vi "Data Processor.vi"(8 "error in (no error)":errorcluster, 11 "Message Queues out":T1) -> (0 "error out":errorcluster, 3 "Message Queue":refnum<queue>)   [LabVIEW 2014]
uses:
  support/Message Queue/All Message Queues.ctl
  support/Message Queue/Message Cluster.ctl
  Data Processor cluster.ctl
  I Adj Parameters.ctl
  Engine/Message.ctl
  Teszt/Teszt.ctl
  Teszt/Command.ctl
  Analog/Enum AO.ctl
  Analog/Enum AI.ctl
  Digital/Enum DO.ctl
  <vilib>/Analysis/baseanly.llb/Mean (DBL).vi
  support/Message Queue/Enqueue Message (Single).vi
  global/Global 1.vi
  <vilib>/Utility/error.llb/Error Cluster From Error Code.vi
  <vilib>/ErrorRing/Error Ring.xnode
  support/Message Queue/Message Queue.lvlib
  Analog/Analog Input Cluster.ctl
  Analog/Analog Result Cluster.ctl
  Analog/Analog data.ctl
  <vilib>/Analysis/NI_AALBase.lvlib
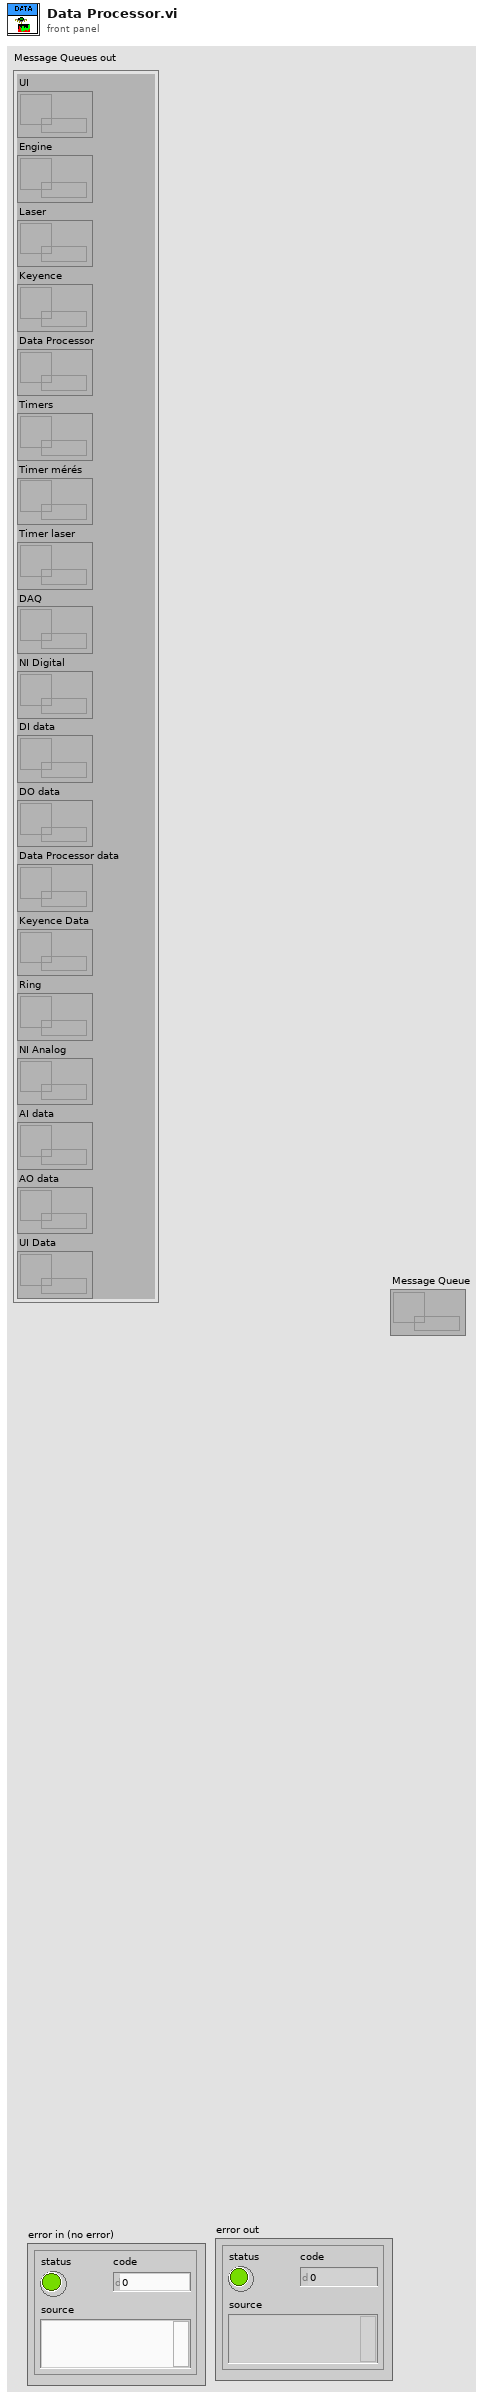
[diagram p1: front panel]
types:
  T1 = typedef "Message Queue.lvlib/All Message Queues.ctl" = cluster{"UI":refnum<queue>, "Engine":refnum<queue>, "Laser":refnum<queue>, "Keyence":refnum<queue>, "Data Processor":refnum<queue>, "Timers":refnum<queue>, "Timer mérés":refnum<queue>, "Timer laser":refnum<queue>, "DAQ":refnum<queue>, "NI Digital":refnum<queue>, "DI data":refnum<queue>, "DO data":refnum<queue>, "Data Processor data":refnum<queue>, "Keyence Data":refnum<queue>, "Ring":refnum<queue>, "NI Analog":refnum<queue>, "AI data":refnum<queue>, "AO data":refnum<queue>, "UI Data":refnum<queue>}
  T2 = typedef "Data Processor cluster.ctl" = cluster{"Dummy":bool, "R Res":dbl, "NTC Res":dbl, "Insulation Res":dbl, "Temperature":dbl, "NTC Exp Res":dbl, "NTC Calc Temp":dbl, "Delta U Puffer":refnum<queue>, "I Adj Parameters":T3, "UCTRL Cluster":cluster{"UCTRL NTC":dbl, "UCTRL R":dbl, "UCTRL dU":dbl}}
  T3 = typedef "I Adj Parameters.ctl" = cluster{"Vr NTC":dbl, "Vr R":dbl, "Vr dU":dbl, "I Adj step":i32, "Output":dbl, "Adj Failed":bool}
  T4 = typedef "Enum AO.ctl" = enum16{"UCTRL"}
  T5 = typedef "Enum AI.ctl" = enum32{"URref", "UR", "UNTC", "UISOL", "TEMP", "dUref", "dU_", "U48"}
  T6 = typedef "Enum DO.ctl" = enum16{"Izolációs relé", "B oldal relé (nincs használva)", "48V relé", "Elszívás KI", "Bördelezés teszt", "Gyûrû megnyomás", "Termék rögzítés", "R mérés relé", "200mA relé", "NTC mérés relé", "Levegõ BE"}
  T7 = typedef "Teszt.ctl" = cluster{"Thread ID":dbl, "Mérésszám":string, "Mérés/Utasítás":string, "Command":T8, "Min":string, "Max":string, "Aktív?":bool, "Log?":bool, "Kiértékelés":bool, "Etalon 1 exp":bool, "Etalon 2 exp":bool, "Etalon 3 exp":bool, "Etalon 4 exp":bool, "Etalon 5 exp":bool}
  T8 = typedef "Command.ctl" = cluster{"Parancs":string, "Paraméter 1":string, "Paraméter 2":string, "Paraméter 3":string, "Paraméter 4":string, "Paraméter 5":string, "Eredmény":string}
  T9 = typedef "Message.ctl" = cluster{"Thread ID":u16, "Callback":string, "Data":variant, "Error":errorcluster}
  T10 = typedef "Analog data.ctl" = cluster{"DAQmx Tasks Started":bool, "Csatorna jellemzõk":T11[], "Delta U Puffer Enable":bool, "Delta U Puffer":refnum<queue>, "URref":refnum<k21>, "UR":refnum<k21>, "UNTC":refnum<k21>, "UISOL":refnum<k21>, "TEMP":refnum<k21>, "dUref":refnum<k21>, "dU_":refnum<k21>, "UCTRL":refnum<k21>, "U48":refnum<k21>, "NI analog":refnum<k21>}
  T11 = typedef "Csatorna jellemzõk.ctl" = cluster{"Név":string, "Átlagolás":i32, "Ritkítás":i32, "Belsõ Puffer":refnum<queue>, "Kimenõ Puffer":refnum<queue>}
  T12 = typedef "Analog Input Cluster.ctl" = cluster{"NI-6221 Continuous Sample":cluster{"Sensor":dbl, "Uref":dbl, "Temperature":dbl, "Uisol":dbl, "NTC":dbl, "U48":dbl, "U15":dbl}, "Analog Result":T13, "NI-6221 N Sample":cluster{"URref":dbl[], "UR":dbl[], "UNTC":dbl[], "UISOL":dbl[], "TEMP":dbl[], "dUref":dbl[], "dU":dbl[], "U48":dbl[]}}
  T13 = typedef "Analog Result Cluster.ctl" = cluster{"Szenzor ellenállás":dbl, "NTC ellenállás":dbl, "Szigetelési ellenállás":dbl, "Hõmérséklet":dbl, "48V":dbl, "15V":dbl, "Elvárt NTC ellenállás":dbl, "Semmi 3":dbl, "Semmi 4":dbl, "Számolt NTC hõmérséklet":dbl}
  T14 = cluster{"[0]":dbl, "[1]":dbl, "[2]":dbl, "[3]":dbl, "[4]":dbl, "[5]":dbl, "[6]":dbl}
  T15 = cluster{"[0]":dbl, "[1]":dbl, "[2]":dbl, "[3]":dbl, "[4]":dbl, "[5]":dbl, "[6]":dbl, "[7]":dbl, "[8]":dbl, "[9]":dbl}
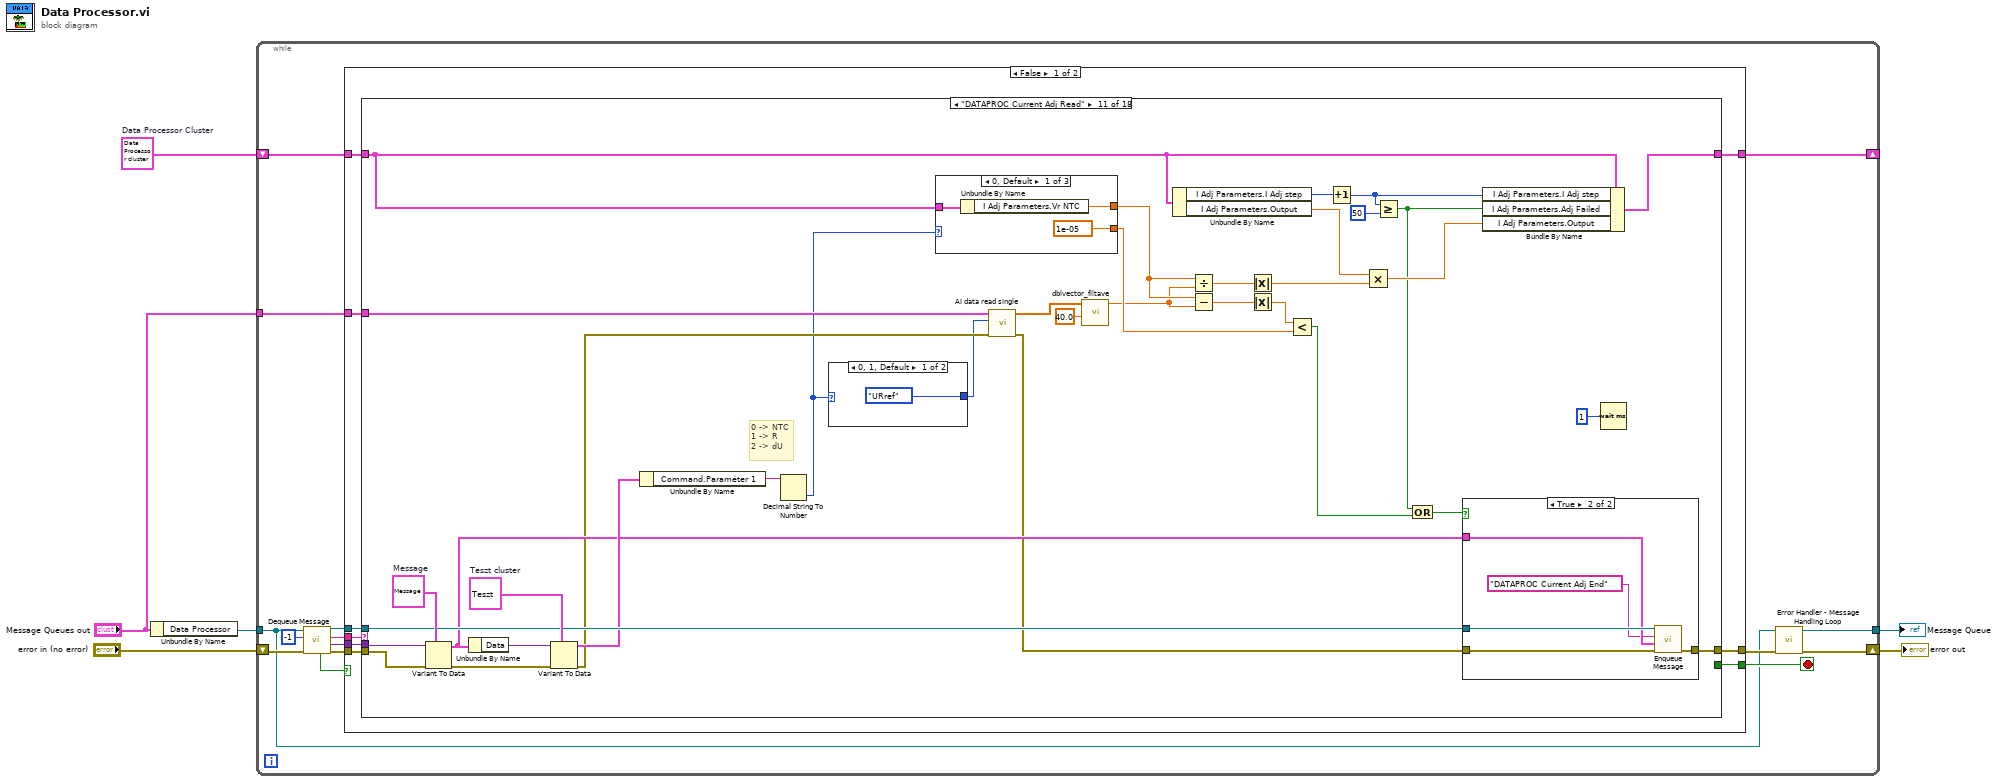
[diagram p0: block diagram]
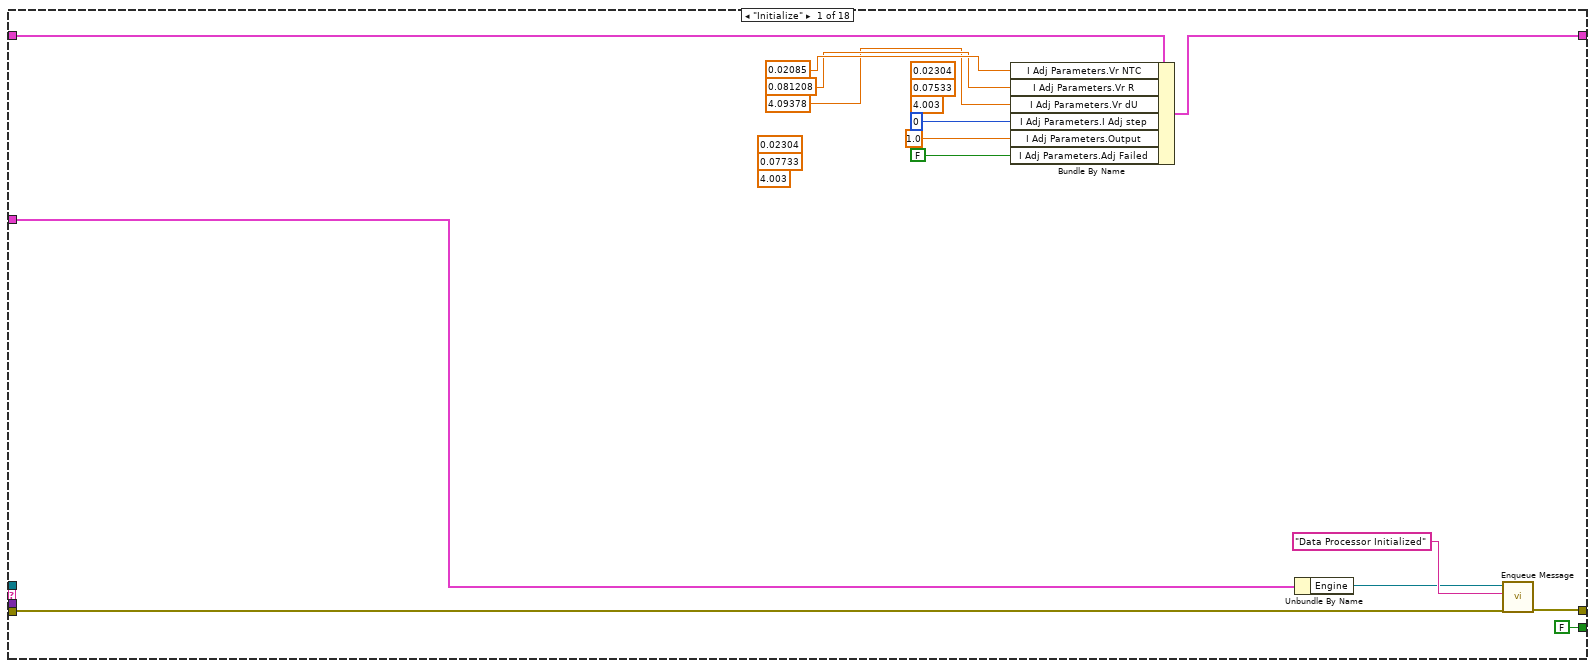
[diagram p2: hidden frame]
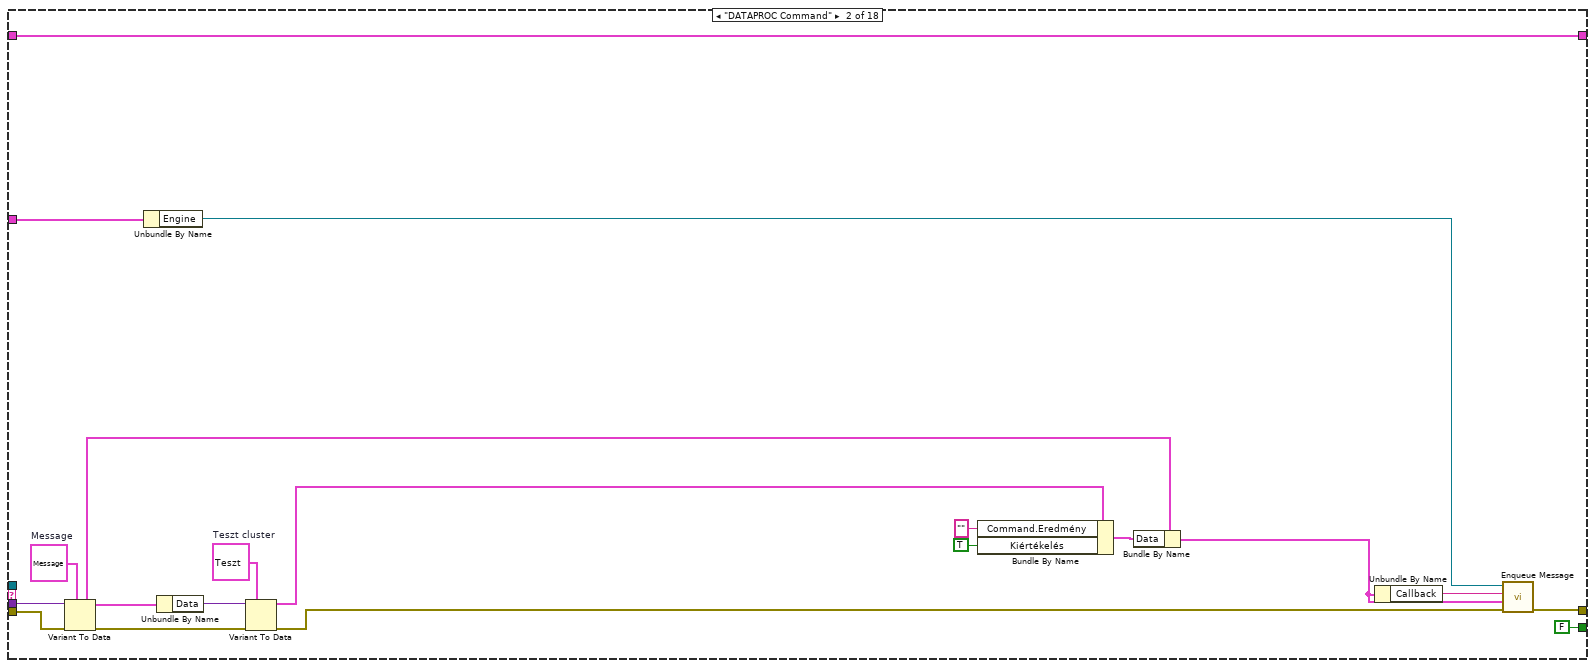
[diagram p3: hidden frame]
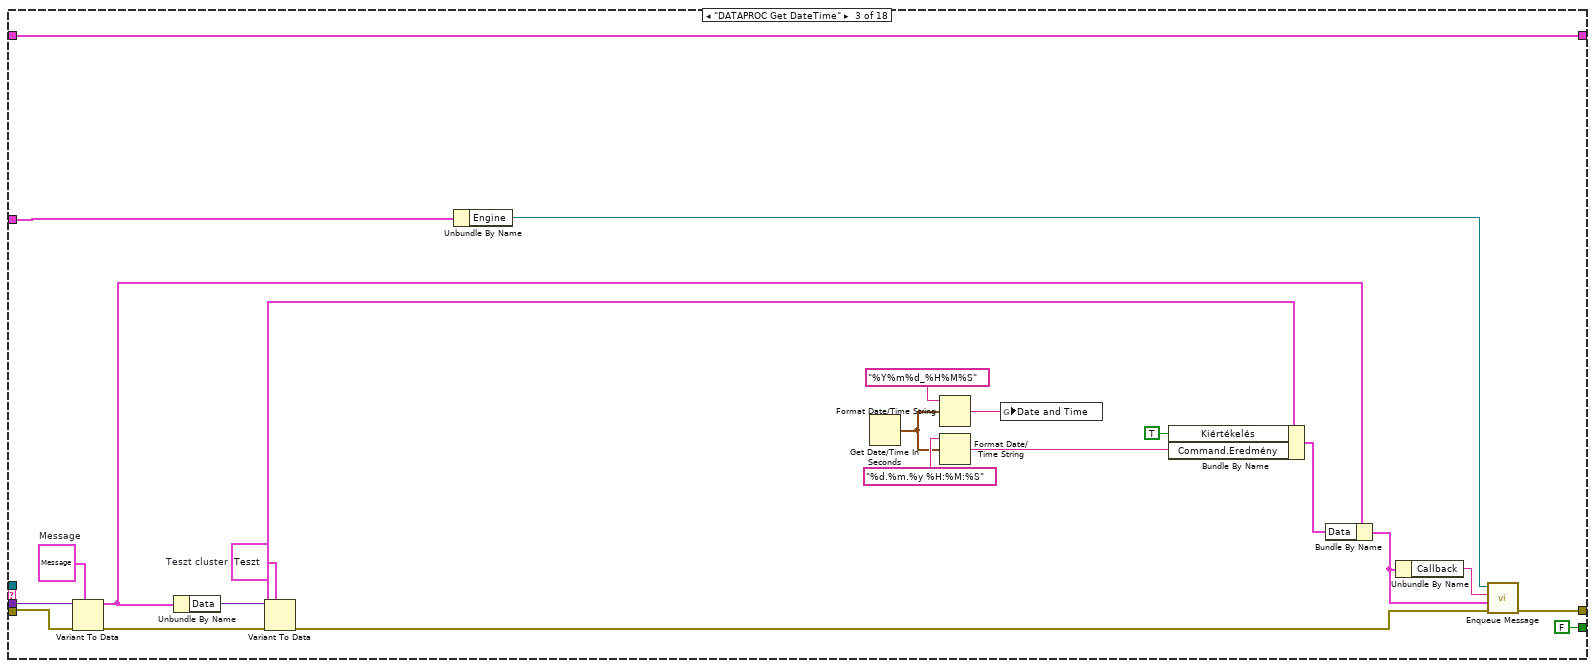
[diagram p4: hidden frame]
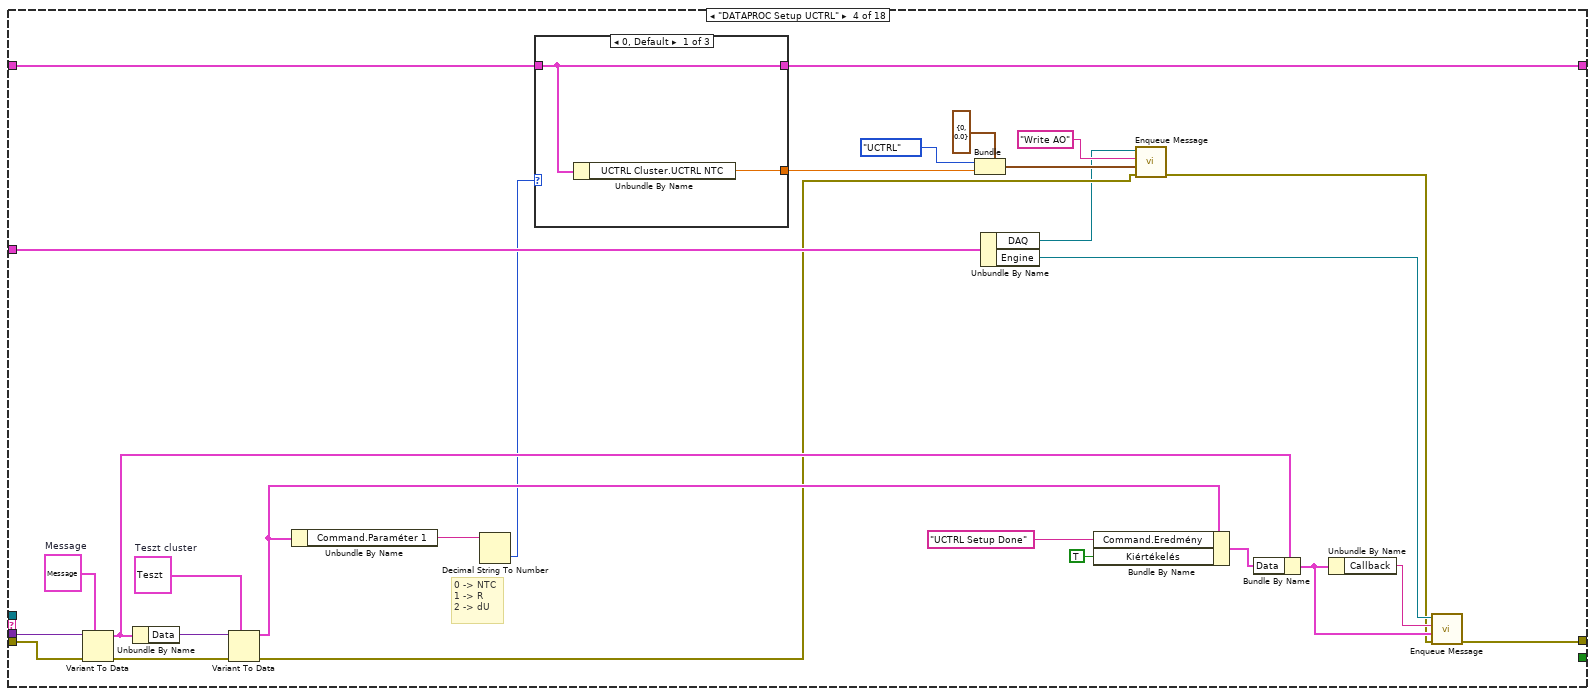
[diagram p5: hidden frame]
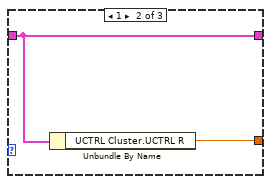
[diagram p6: hidden frame]
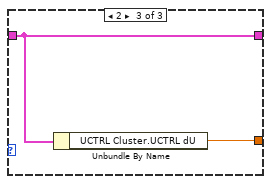
[diagram p7: hidden frame]
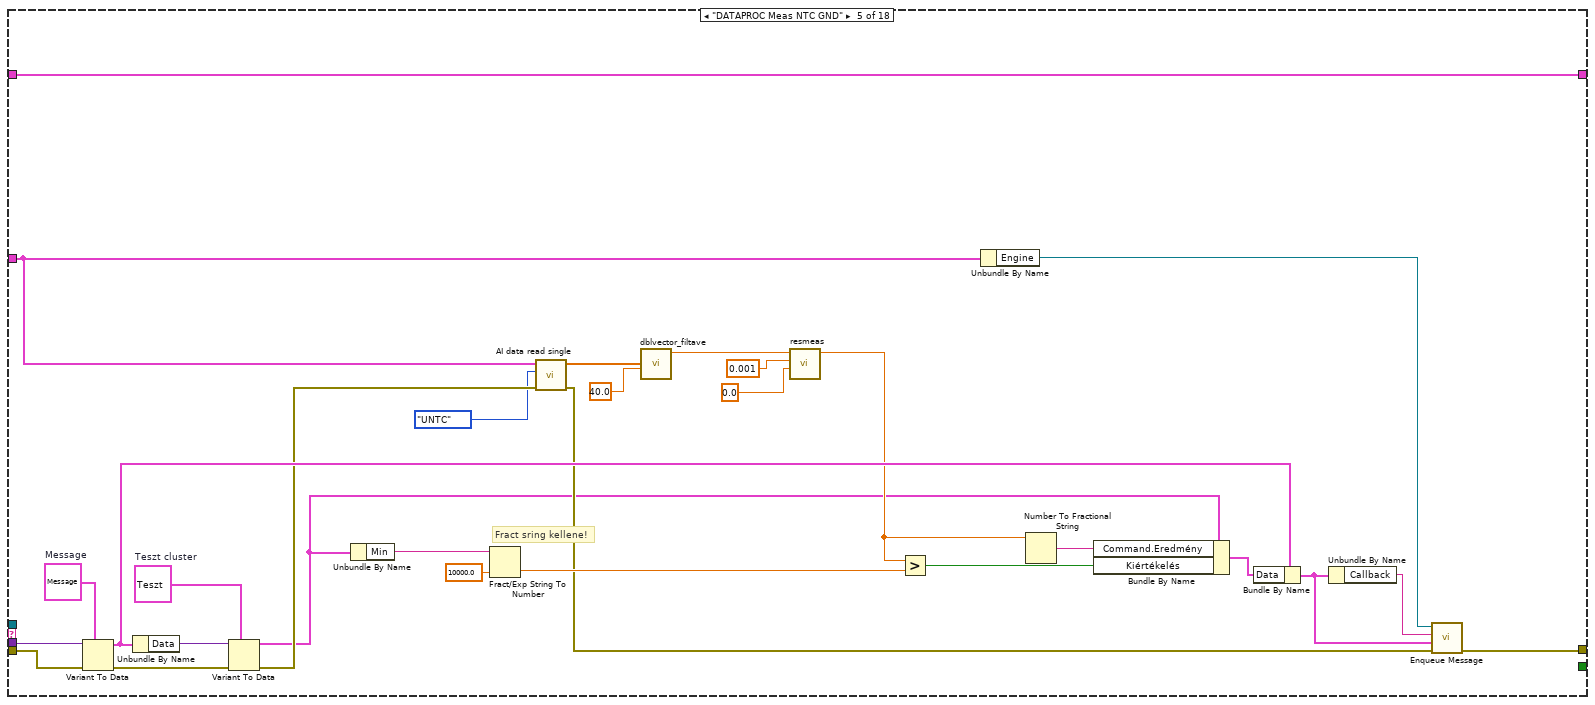
[diagram p8: hidden frame]
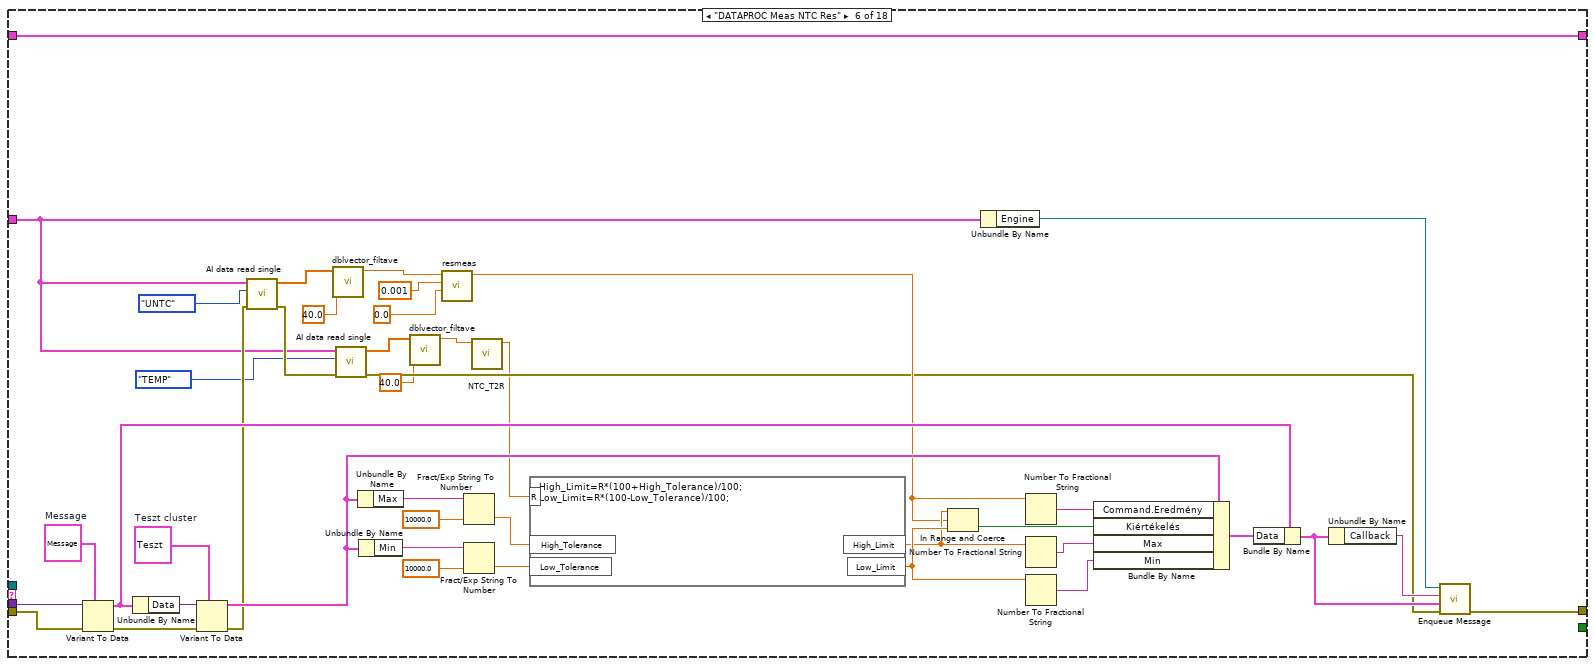
[diagram p9: hidden frame]
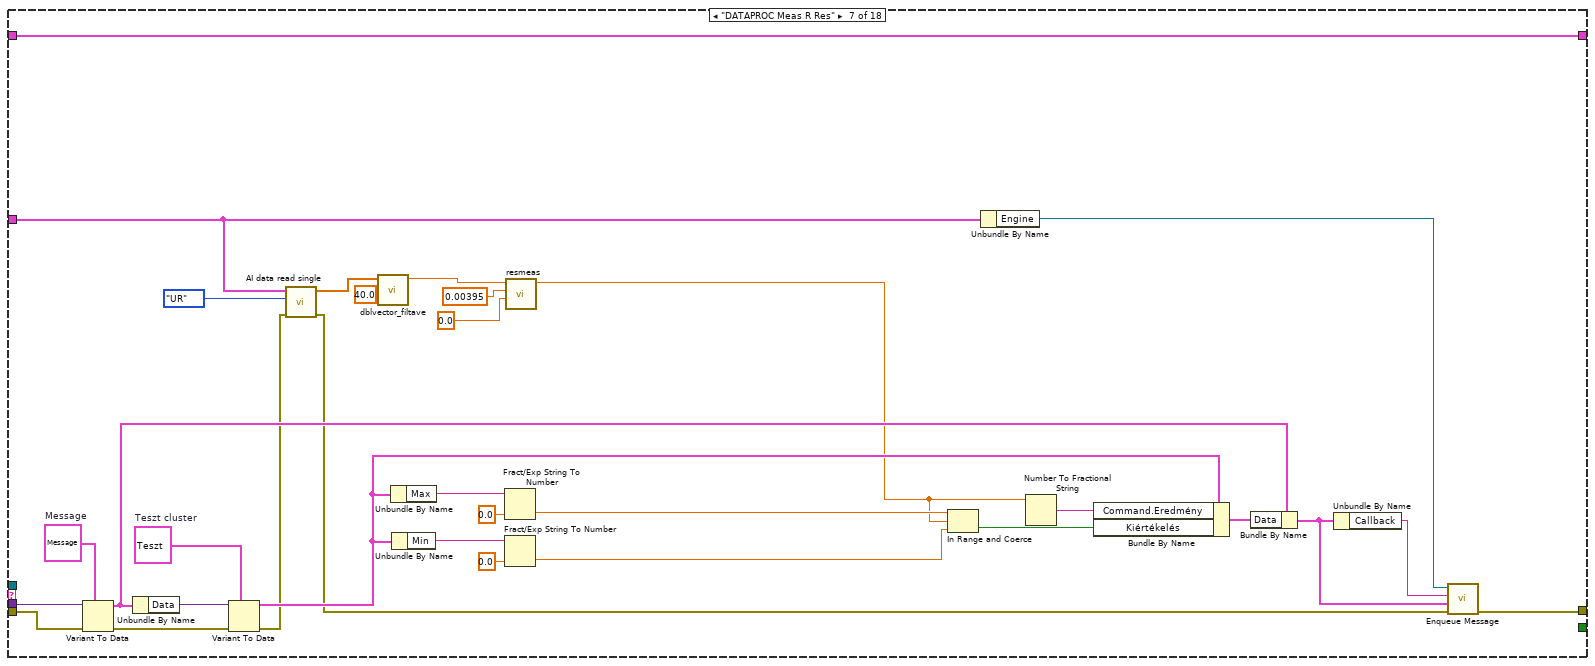
[diagram p10: hidden frame]
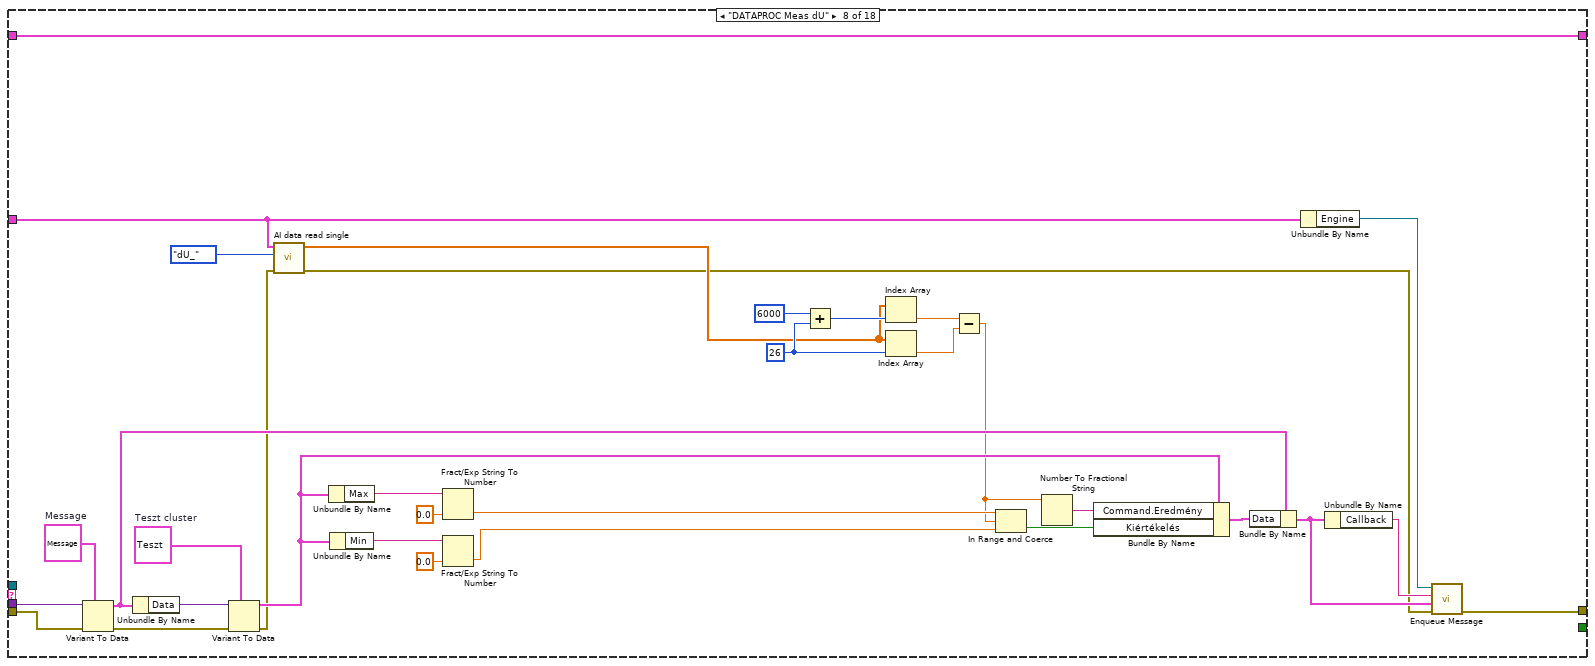
[diagram p11: hidden frame]
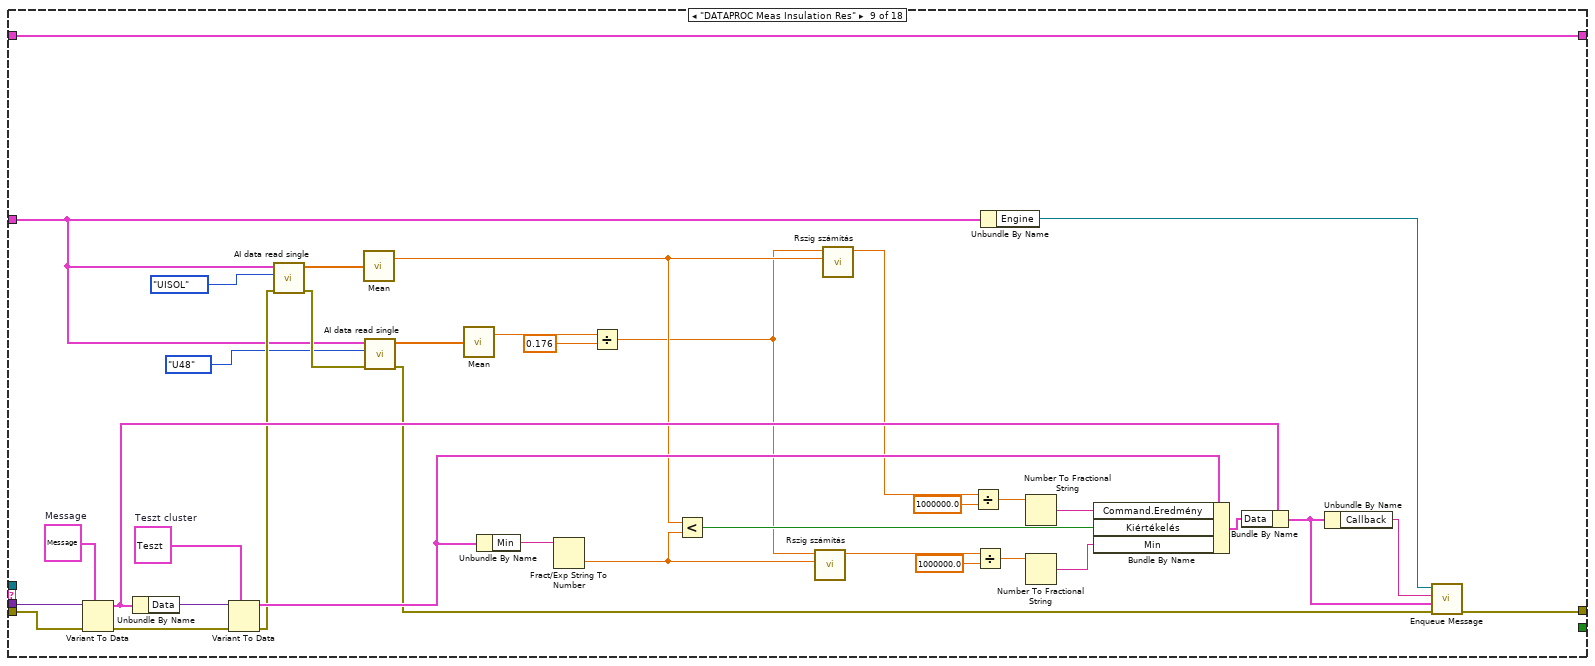
[diagram p12: hidden frame]
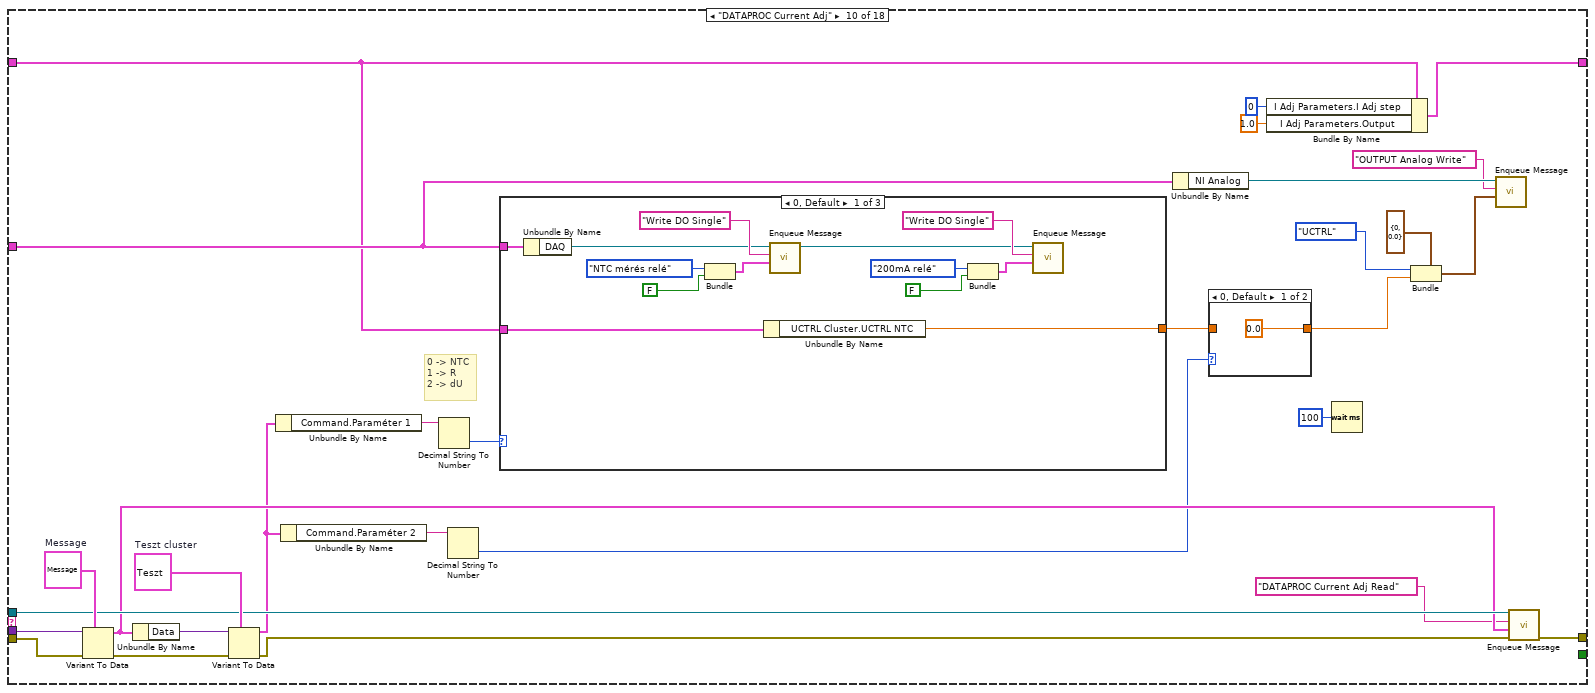
[diagram p13: hidden frame]
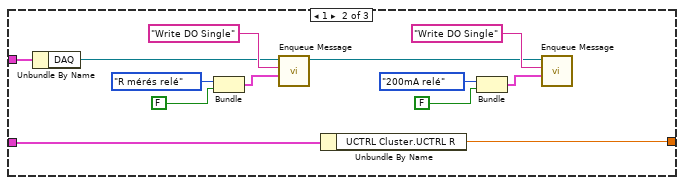
[diagram p15: hidden frame]
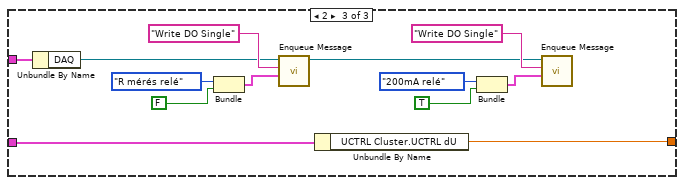
[diagram p16: hidden frame]
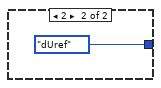
[diagram p17: hidden frame]
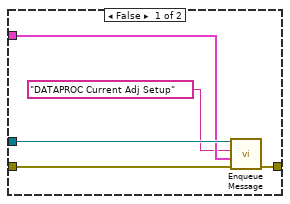
[diagram p18: hidden frame]
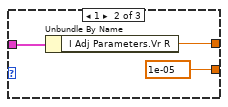
[diagram p19: hidden frame]
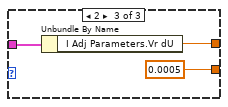
[diagram p20: hidden frame]
diagram:
  w1 = T2 {"Dummy"=FALSE, "R Res"=0.0, "NTC Res"=0.0, "Insulation Res"=0.0, "Temperature"=0.0, "NTC Exp Res"=0.0, "NTC Calc Temp"=0.0, "Delta U Puffer"=refnum, "I Adj Parameters"={"Vr NTC"=0.0, "Vr R"=0.0, "Vr dU"=0.0, "I Adj step"=0, "Output"=0.0, "Adj Failed"=FALSE}, "UCTRL Cluster"={"UCTRL NTC"=0.0, "UCTRL R"=0.0, "UCTRL dU"=0.0}}  # Data Processor Cluster
  n1 = Unbundle By Name("Message Queues out") -> ("Data Processor"=w3:refnum<queue>)
  n2 = while {
    tunnel: w3 -> [w7]
    shift-right: [w8] -> _
    shift-left: w1 -> [w14]
    shift-right: [w12] -> w6
    shift-left: "error in (no error)" -> [w21]
    tunnel: "Message Queues out" -> [w10]
    tunnel: [w9] -> w2
    stop <- w17 stop-if-true
    n3 = call "Dequeue Message.vi"("error in (no error)"=w21, "timeout in ms (-1)"=-1, "Message Queue"=w7) -> ("error out"=w19:errorcluster, "Message Data"=w13:variant, "Message"=w20:string, "dup Message Queue"=w18:refnum<queue>, "timed out?"=w15:bool)  [unwired: 4 in]
    n4 = case shown="False" w15 {
      tunnel: w20 -> [w30 _]
      tunnel: w19 -> [w29 w565]
      tunnel: w18 -> [w28 _]
      tunnel: [w27 FALSE] -> w17
      tunnel: [w26 w564] -> w11
      tunnel: w14 -> [w24 w563]
      tunnel: [w25 w562] -> w8
      tunnel: w13 -> [w23 _]
      tunnel: w10 -> [w22 w566]
      frame False {
        n5 = case shown="\"DATAPROC Current Adj Read\"" w30 {
          selector: w30 -> [_ _ _ _ _ _ _ _ _ _ _ _ _ _ _ _ _ w551]
          tunnel: w29 -> [w39 w55 w85 w107 w142 w184 w216 w249 w286 w317 w394 w443 w471 w521 w523 w537 w540 _]
          tunnel: w28 -> [_ _ _ _ _ _ _ _ _ w314 w392 w441 _ w520 w526 w536 w550 _]
          tunnel: [w43 w62 w77 w109 w144 w186 w218 w251 w288 w316 w393 w442 w473 w518 w527 w538 w541 w552] -> w26
          tunnel: [FALSE FALSE FALSE _ _ _ _ _ _ _ _ _ _ _ _ _ TRUE FALSE] -> w27
          tunnel: [w37 w45 w83 w90 w141 w183 w215 w248 w285 w309 w373 w422 w461 w519 w522 w539 w548 w554] -> w25
          tunnel: w24 -> [w38 w45 w83 w91 w141 w183 w215 w248 w285 w295 w374 w423 w456 w519 w522 w539 w548 w554]
          tunnel: w23 -> [_ w54 w84 w108 w143 w185 w217 w250 w287 w318 w395 w444 w472 _ w524 _ _ _]
          tunnel: w22 -> [w40 w60 w78 w94 w131 w155 w203 w239 w266 w305 w370 w439 w454 _ w525 _ w543 _]
          frame "Initialize" {
            (unwired) 4.003 ("I Adj Parameters.Vr dU")
            (unwired) 0.07733 ("I Adj Parameters.Vr R")
            (unwired) 0.02304 ("I Adj Parameters.Vr NTC")
            (unwired) 4.003 ("I Adj Parameters.Vr dU")
            (unwired) 0.07533 ("I Adj Parameters.Vr R")
            (unwired) 0.02304 ("I Adj Parameters.Vr NTC")
            n6 = Bundle By Name(cluster=w38, "I Adj Parameters.Vr NTC"=0.02085, "I Adj Parameters.Vr R"=0.081208, "I Adj Parameters.Vr dU"=4.09378, "I Adj Parameters.I Adj step"=0, "I Adj Parameters.Output"=1.0, "I Adj Parameters.Adj Failed"=FALSE) -> (w37:T2)
            n7 = Unbundle By Name(w40) -> ("Engine"=w41:refnum<queue>)
            n8 = call-poly "Enqueue Message.vi"("error in (no error)"=w39, "Message"="Data Processor Initialized", "Message Queue"=w41) -> ("error out"=w43:errorcluster)  [unwired: 7 in, 1 out]
          }
          frame "DATAPROC Command" {
            w56 = T7 {"Thread ID"=0.0, "Mérésszám"="", "Mérés/Utasítás"="", "Command"={"Parancs"="", "Paraméter 1"="", "Paraméter 2"="", "Paraméter 3"="", "Paraméter 4"="", "Paraméter 5"="", "Eredmény"=""}, "Min"="", "Max"="", "Aktív?"=FALSE, "Log?"=FALSE, "Kiértékelés"=FALSE, "Etalon 1 exp"=FALSE, "Etalon 2 exp"=FALSE, "Etalon 3 exp"=FALSE, "Etalon 4 exp"=FALSE, "Etalon 5 exp"=FALSE}  # Teszt cluster
            w59 = T9 {"Thread ID"=0, "Callback"="", "Data"=variant, "Error"={"status"=FALSE, "code"=0, "source"=""}}  # Message
            n9 = Variant To Data(error in=w55, type=w59, Variant=w54) -> (data=w50:T9, error out=w58:errorcluster)
            n10 = Unbundle By Name(w60) -> ("Engine"=w61:refnum<queue>)
            n11 = Unbundle By Name(w50) -> ("Data"=w57:variant)
            n12 = Variant To Data(error in=w58, type=w56, Variant=w57) -> (data=w46:T7, error out=w49:errorcluster)
            n13 = Bundle By Name(cluster=w46, "Command.Eredmény"="", "Kiértékelés"=TRUE) -> (w53:T7)
            n14 = Bundle By Name(cluster=w50, "Data"=w53) -> (w51:T9)
            n15 = Unbundle By Name(w51) -> ("Callback"=w52:string)
            n16 = call-poly "Enqueue Message.vi"("error in (no error)"=w49, "Message Data"=w51, "Message"=w52, "Message Queue"=w61) -> ("error out"=w62:errorcluster)  [unwired: 6 in, 1 out]
          }
          frame "DATAPROC Get DateTime" {
            w79 = T7 {"Thread ID"=0.0, "Mérésszám"="", "Mérés/Utasítás"="", "Command"={"Parancs"="", "Paraméter 1"="", "Paraméter 2"="", "Paraméter 3"="", "Paraméter 4"="", "Paraméter 5"="", "Eredmény"=""}, "Min"="", "Max"="", "Aktív?"=FALSE, "Log?"=FALSE, "Kiértékelés"=FALSE, "Etalon 1 exp"=FALSE, "Etalon 2 exp"=FALSE, "Etalon 3 exp"=FALSE, "Etalon 4 exp"=FALSE, "Etalon 5 exp"=FALSE}  # Teszt cluster
            w82 = T9 {"Thread ID"=0, "Callback"="", "Data"=variant, "Error"={"status"=FALSE, "code"=0, "source"=""}}  # Message
            n17 = Variant To Data(error in=w85, type=w82, Variant=w84) -> (data=w73:T9, error out=w81:errorcluster)
            n18 = Unbundle By Name(w73) -> ("Data"=w80:variant)
            n19 = Variant To Data(error in=w81, type=w79, Variant=w80) -> (data=w70:T7, error out=w71:errorcluster)
            n20 = Unbundle By Name(w78) -> ("Engine"=w76:refnum<queue>)
            n21 = Get Date/Time In Seconds() -> (seconds since 1Jan1904=w66:timestamp)
            n22 = Format Date/Time String(time format string (%c)="%Y%m%d_%H%M%S", seconds (now)=w66) -> (date/time string=w64:string)  [unwired: 1 in]
            n23 = Format Date/Time String(time format string (%c)="%d.%m.%y %H:%M:%S", seconds (now)=w66) -> (date/time string=w68:string)  [unwired: 1 in]
            n24 = global write "Global 1.vi" "Date and Time"(w64) -> ()
            n25 = Bundle By Name(cluster=w70, "Kiértékelés"=TRUE, "Command.Eredmény"=w68) -> (w75:T7)
            n26 = Bundle By Name(cluster=w73, "Data"=w75) -> (w72:T9)
            n27 = Unbundle By Name(w72) -> ("Callback"=w74:string)
            n28 = call-poly "Enqueue Message.vi"("error in (no error)"=w71, "Message Data"=w72, "Message"=w74, "Message Queue"=w76) -> ("error out"=w77:errorcluster)  [unwired: 6 in, 1 out]
          }
          frame "DATAPROC Setup UCTRL" {
            w113 = T9 {"Thread ID"=0, "Callback"="", "Data"=variant, "Error"={"status"=FALSE, "code"=0, "source"=""}}  # Message
            w110 = T7 {"Thread ID"=0.0, "Mérésszám"="", "Mérés/Utasítás"="", "Command"={"Parancs"="", "Paraméter 1"="", "Paraméter 2"="", "Paraméter 3"="", "Paraméter 4"="", "Paraméter 5"="", "Eredmény"=""}, "Min"="", "Max"="", "Aktív?"=FALSE, "Log?"=FALSE, "Kiértékelés"=FALSE, "Etalon 1 exp"=FALSE, "Etalon 2 exp"=FALSE, "Etalon 3 exp"=FALSE, "Etalon 4 exp"=FALSE, "Etalon 5 exp"=FALSE}  # Teszt cluster
            # "0 -> NTC\n1 -> R\n2 -> dU"
            n29 = Variant To Data(error in=w107, type=w113, Variant=w108) -> (data=w114:T9, error out=w111:errorcluster)
            n30 = Unbundle By Name(w114) -> ("Data"=w112:variant)
            n31 = Variant To Data(error in=w111, type=w110, Variant=w112) -> (data=w102:T7, error out=w89:errorcluster)
            n32 = Unbundle By Name(w102) -> ("Command.Paraméter 1"=w101:string)
            n33 = Decimal String To Number(string=w101) -> (number=w92:i32)  [unwired: 2 in, 1 out]
            n34 = case shown="0, Default" w92 {
              tunnel: [w116 w118 w120] -> w93
              tunnel: w91 -> [w115 w117 w119]
              tunnel: [w115 w117 w119] -> w90
              frame 0, Default {
                n35 = Unbundle By Name(w115) -> ("UCTRL Cluster.UCTRL NTC"=w116:dbl)
              }
              frame 1 {
                n36 = Unbundle By Name(w117) -> ("UCTRL Cluster.UCTRL R"=w118:dbl)
              }
              frame 2 {
                n37 = Unbundle By Name(w119) -> ("UCTRL Cluster.UCTRL dU"=w120:dbl)
              }
            }
            n38 = Bundle(cluster=cluster{i32, "UCtrl":dbl} {0, "UCtrl"=0.0}, Enum_AO."UCTRL" ("Enum"), "UCtrl"=w93) -> (w98:cluster{i32, "UCtrl":dbl})
            n39 = Unbundle By Name(w94) -> ("DAQ"=w87:refnum<queue>, "Engine"=w103:refnum<queue>)
            n40 = Bundle By Name(cluster=w102, "Command.Eredmény"="UCTRL Setup Done", "Kiértékelés"=TRUE) -> (w106:T7)
            n41 = call-poly "Enqueue Message.vi"("error in (no error)"=w89, "Message Data"=w98, "Message"="Write AO", "Message Queue"=w87) -> ("error out"=w88:errorcluster)  [unwired: 6 in, 1 out]
            n42 = Bundle By Name(cluster=w114, "Data"=w106) -> (w104:T9)
            n43 = Unbundle By Name(w104) -> ("Callback"=w105:string)
            n44 = call-poly "Enqueue Message.vi"("error in (no error)"=w88, "Message Data"=w104, "Message"=w105, "Message Queue"=w103) -> ("error out"=w109:errorcluster)  [unwired: 6 in, 1 out]
          }
          frame "DATAPROC Meas NTC GND" {
            w148 = T9 {"Thread ID"=0, "Callback"="", "Data"=variant, "Error"={"status"=FALSE, "code"=0, "source"=""}}  # Message
            w145 = T7 {"Thread ID"=0.0, "Mérésszám"="", "Mérés/Utasítás"="", "Command"={"Parancs"="", "Paraméter 1"="", "Paraméter 2"="", "Paraméter 3"="", "Paraméter 4"="", "Paraméter 5"="", "Eredmény"=""}, "Min"="", "Max"="", "Aktív?"=FALSE, "Log?"=FALSE, "Kiértékelés"=FALSE, "Etalon 1 exp"=FALSE, "Etalon 2 exp"=FALSE, "Etalon 3 exp"=FALSE, "Etalon 4 exp"=FALSE, "Etalon 5 exp"=FALSE}  # Teszt cluster
            # "Fract sring kellene!"
            n45 = Variant To Data(error in=w142, type=w148, Variant=w143) -> (data=w149:T9, error out=w146:errorcluster)
            n46 = Unbundle By Name(w149) -> ("Data"=w147:variant)
            n47 = Variant To Data(error in=w146, type=w145, Variant=w147) -> (data=w123:T7, error out=w130:errorcluster)
            n48 = Unbundle By Name(w123) -> ("Min"=w134:string)
            n49 = Fract/Exp String To Number(string=w134, default (0 dbl)=10000.0 ("NTC Res")) -> (number=w132:dbl)  [unwired: 2 in, 1 out]
            n50 = call "AI data read single.vi"("error in (no error)"=w130, "Numeric"=Enum_AI."UNTC" ("Message"), "Message Queues in"=w131) -> ("error out"=w129:errorcluster, "Array"=w126:dbl[])  [unwired: 7 in]
            n51 = call "dblvector_filtave.vi"("Eldobandó [%]"=40.0, "Mérési adatok"=w126) -> ("Szûrt átlag"=w125:dbl)  [unwired: 9 in]
            n52 = call "resmeas.vi"("Rc"=0.0, "Im"=0.001, "Um"=w125) -> ("Rm"=w124:dbl)  [unwired: 8 in]
            n53 = Greater?(x=w124, y=w132) -> (0:w136:bool)
            n54 = Unbundle By Name(w131) -> ("Engine"=w137:refnum<queue>)
            n55 = Number To Fractional String(number=w124) -> (F-format string=w135:string)  [unwired: 3 in]
            n56 = Bundle By Name(cluster=w123, "Command.Eredmény"=w135, "Kiértékelés"=w136) -> (w140:T7)
            n57 = Bundle By Name(cluster=w149, "Data"=w140) -> (w138:T9)
            n58 = Unbundle By Name(w138) -> ("Callback"=w139:string)
            n59 = call-poly "Enqueue Message.vi"("error in (no error)"=w129, "Message Data"=w138, "Message"=w139, "Message Queue"=w137) -> ("error out"=w144:errorcluster)  [unwired: 6 in, 1 out]
          }
          frame "DATAPROC Meas NTC Res" {
            w190 = T9 {"Thread ID"=0, "Callback"="", "Data"=variant, "Error"={"status"=FALSE, "code"=0, "source"=""}}  # Message
            w187 = T7 {"Thread ID"=0.0, "Mérésszám"="", "Mérés/Utasítás"="", "Command"={"Parancs"="", "Paraméter 1"="", "Paraméter 2"="", "Paraméter 3"="", "Paraméter 4"="", "Paraméter 5"="", "Eredmény"=""}, "Min"="", "Max"="", "Aktív?"=FALSE, "Log?"=FALSE, "Kiértékelés"=FALSE, "Etalon 1 exp"=FALSE, "Etalon 2 exp"=FALSE, "Etalon 3 exp"=FALSE, "Etalon 4 exp"=FALSE, "Etalon 5 exp"=FALSE}  # Teszt cluster
            n60 = Variant To Data(error in=w184, type=w190, Variant=w185) -> (data=w191:T9, error out=w188:errorcluster)
            n61 = Unbundle By Name(w191) -> ("Data"=w189:variant)
            n62 = Variant To Data(error in=w188, type=w187, Variant=w189) -> (data=w168:T7, error out=w165:errorcluster)
            n63 = call "AI data read single.vi"("error in (no error)"=w165, "Numeric"=Enum_AI."UNTC" ("Message"), "Message Queues in"=w155) -> ("error out"=w158:errorcluster, "Array"=w161:dbl[])  [unwired: 7 in]
            n64 = call "dblvector_filtave.vi"("Eldobandó [%]"=40.0, "Mérési adatok"=w161) -> ("Szûrt átlag"=w162:dbl)  [unwired: 9 in]
            n65 = call "AI data read single.vi"("error in (no error)"=w158, "Numeric"=Enum_AI."TEMP" ("Message"), "Message Queues in"=w155) -> ("error out"=w157:errorcluster, "Array"=w154:dbl[])  [unwired: 7 in]
            n66 = Unbundle By Name(w168) -> ("Max"=w172:string)
            n67 = Unbundle By Name(w168) -> ("Min"=w170:string)
            n68 = call "dblvector_filtave.vi"("Eldobandó [%]"=40.0, "Mérési adatok"=w154) -> ("Szûrt átlag"=w153:dbl)  [unwired: 9 in]
            n69 = call "resmeas.vi"("Rc"=0.0, "Im"=0.001, "Um"=w162) -> ("Rm"=w159:dbl)  [unwired: 8 in]
            n70 = Fract/Exp String To Number(string=w172, default (0 dbl)=10000.0 ("NTC Res")) -> (number=w167:dbl)  [unwired: 2 in, 1 out]
            n71 = Fract/Exp String To Number(string=w170, default (0 dbl)=10000.0 ("NTC Res")) -> (number=w166:dbl)  [unwired: 2 in, 1 out]
            n72 = call "NTC_T2R.vi"("Temperature"=w153) -> ("Resistance"=w152:dbl)  [unwired: 10 in]
            n73 = formula code="High_Limit=R*(100+High_Tolerance)/100;\nLow_Limit=R*(100-Low_Tolerance)/100;"("High_Tolerance"=w167, "Low_Tolerance"=w166, "R"=w152) -> ("High_Limit"=w181:dbl, "Low_Limit"=w182:dbl)
            n74 = In Range and Coerce(upper limit=w181, x=w159, lower limit=w182) -> (In Range?=w176:bool)  [unwired: 1 out]
            n75 = Unbundle By Name(w155) -> ("Engine"=w177:refnum<queue>)
            n76 = Number To Fractional String(number=w159) -> (F-format string=w175:string)  [unwired: 3 in]
            n77 = Number To Fractional String(number=w181) -> (F-format string=w174:string)  [unwired: 3 in]
            n78 = Number To Fractional String(number=w182) -> (F-format string=w173:string)  [unwired: 3 in]
            n79 = Bundle By Name(cluster=w168, "Command.Eredmény"=w175, "Kiértékelés"=w176, "Max"=w174, "Min"=w173) -> (w180:T7)
            n80 = Bundle By Name(cluster=w191, "Data"=w180) -> (w178:T9)
            n81 = Unbundle By Name(w178) -> ("Callback"=w179:string)
            n82 = call-poly "Enqueue Message.vi"("error in (no error)"=w157, "Message Data"=w178, "Message"=w179, "Message Queue"=w177) -> ("error out"=w186:errorcluster)  [unwired: 6 in, 1 out]
          }
          frame "DATAPROC Meas R Res" {
            w222 = T9 {"Thread ID"=0, "Callback"="", "Data"=variant, "Error"={"status"=FALSE, "code"=0, "source"=""}}  # Message
            w219 = T7 {"Thread ID"=0.0, "Mérésszám"="", "Mérés/Utasítás"="", "Command"={"Parancs"="", "Paraméter 1"="", "Paraméter 2"="", "Paraméter 3"="", "Paraméter 4"="", "Paraméter 5"="", "Eredmény"=""}, "Min"="", "Max"="", "Aktív?"=FALSE, "Log?"=FALSE, "Kiértékelés"=FALSE, "Etalon 1 exp"=FALSE, "Etalon 2 exp"=FALSE, "Etalon 3 exp"=FALSE, "Etalon 4 exp"=FALSE, "Etalon 5 exp"=FALSE}  # Teszt cluster
            n83 = Variant To Data(error in=w216, type=w222, Variant=w217) -> (data=w223:T9, error out=w220:errorcluster)
            n84 = Unbundle By Name(w223) -> ("Data"=w221:variant)
            n85 = Variant To Data(error in=w220, type=w219, Variant=w221) -> (data=w204:T7, error out=w202:errorcluster)
            n86 = call "AI data read single.vi"("error in (no error)"=w202, "Numeric"=Enum_AI."UR" ("Message"), "Message Queues in"=w203) -> ("error out"=w201:errorcluster, "Array"=w195:dbl[])  [unwired: 7 in]
            n87 = call "dblvector_filtave.vi"("Eldobandó [%]"=40.0, "Mérési adatok"=w195) -> ("Szûrt átlag"=w194:dbl)  [unwired: 9 in]
            n88 = Unbundle By Name(w204) -> ("Max"=w208:string)
            n89 = Unbundle By Name(w204) -> ("Min"=w207:string)
            n90 = Fract/Exp String To Number(string=w208, default (0 dbl)=0.0 ("default (0 I32)")) -> (number=w206:dbl)  [unwired: 2 in, 1 out]
            n91 = Fract/Exp String To Number(string=w207, default (0 dbl)=0.0 ("default (0 I32)")) -> (number=w205:dbl)  [unwired: 2 in, 1 out]
            n92 = call "resmeas.vi"("Rc"=0.0, "Im"=0.00395, "Um"=w194) -> ("Rm"=w193:dbl)  [unwired: 8 in]
            n93 = In Range and Coerce(upper limit=w206, x=w193, lower limit=w205) -> (In Range?=w210:bool)  [unwired: 1 out]
            n94 = Unbundle By Name(w203) -> ("Engine"=w211:refnum<queue>)
            n95 = Number To Fractional String(number=w193) -> (F-format string=w209:string)  [unwired: 3 in]
            n96 = Bundle By Name(cluster=w204, "Command.Eredmény"=w209, "Kiértékelés"=w210) -> (w214:T7)
            n97 = Bundle By Name(cluster=w223, "Data"=w214) -> (w212:T9)
            n98 = Unbundle By Name(w212) -> ("Callback"=w213:string)
            n99 = call-poly "Enqueue Message.vi"("error in (no error)"=w201, "Message Data"=w212, "Message"=w213, "Message Queue"=w211) -> ("error out"=w218:errorcluster)  [unwired: 6 in, 1 out]
          }
          frame "DATAPROC Meas dU" {
            w227 = 26 ("index")
            w255 = T9 {"Thread ID"=0, "Callback"="", "Data"=variant, "Error"={"status"=FALSE, "code"=0, "source"=""}}  # Message
            w252 = T7 {"Thread ID"=0.0, "Mérésszám"="", "Mérés/Utasítás"="", "Command"={"Parancs"="", "Paraméter 1"="", "Paraméter 2"="", "Paraméter 3"="", "Paraméter 4"="", "Paraméter 5"="", "Eredmény"=""}, "Min"="", "Max"="", "Aktív?"=FALSE, "Log?"=FALSE, "Kiértékelés"=FALSE, "Etalon 1 exp"=FALSE, "Etalon 2 exp"=FALSE, "Etalon 3 exp"=FALSE, "Etalon 4 exp"=FALSE, "Etalon 5 exp"=FALSE}  # Teszt cluster
            n100 = Variant To Data(error in=w249, type=w255, Variant=w250) -> (data=w256:T9, error out=w253:errorcluster)
            n101 = Unbundle By Name(w256) -> ("Data"=w254:variant)
            n102 = Variant To Data(error in=w253, type=w252, Variant=w254) -> (data=w245:T7, error out=w240:errorcluster)
            n103 = call "AI data read single.vi"("error in (no error)"=w240, "Numeric"=Enum_AI."dU_" ("Message"), "Message Queues in"=w239) -> ("error out"=w224:errorcluster, "Array"=w225:dbl[])  [unwired: 7 in]
            n104 = Unbundle By Name(w245) -> ("Max"=w247:string)
            n105 = Unbundle By Name(w245) -> ("Min"=w246:string)
            n106 = Fract/Exp String To Number(string=w247, default (0 dbl)=0.0 ("default (0 I32)")) -> (number=w244:dbl)  [unwired: 2 in, 1 out]
            n107 = Fract/Exp String To Number(string=w246, default (0 dbl)=0.0 ("default (0 I32)")) -> (number=w243:dbl)  [unwired: 2 in, 1 out]
            n108 = Add(x=6000, y=w227) -> (x+y=w226:i32)
            n109 = Index Array(array=w225, index=w226) -> (element=w230:dbl)
            n110 = Index Array(array=w225, index=w227) -> (element=w228:dbl)
            n111 = Subtract(x=w230, y=w228) -> (x-y=w229:dbl)
            n112 = In Range and Coerce(upper limit=w244, x=w229, lower limit=w243) -> (In Range?=w233:bool)  [unwired: 1 out]
            n113 = Number To Fractional String(number=w229) -> (F-format string=w232:string)  [unwired: 3 in]
            n114 = Bundle By Name(cluster=w245, "Command.Eredmény"=w232, "Kiértékelés"=w233) -> (w237:T7)
            n115 = Bundle By Name(cluster=w256, "Data"=w237) -> (w235:T9)
            n116 = Unbundle By Name(w239) -> ("Engine"=w234:refnum<queue>)
            n117 = Unbundle By Name(w235) -> ("Callback"=w236:string)
            n118 = call-poly "Enqueue Message.vi"("error in (no error)"=w224, "Message Data"=w235, "Message"=w236, "Message Queue"=w234) -> ("error out"=w251:errorcluster)  [unwired: 6 in, 1 out]
          }
          frame "DATAPROC Meas Insulation Res" {
            w292 = T9 {"Thread ID"=0, "Callback"="", "Data"=variant, "Error"={"status"=FALSE, "code"=0, "source"=""}}  # Message
            w289 = T7 {"Thread ID"=0.0, "Mérésszám"="", "Mérés/Utasítás"="", "Command"={"Parancs"="", "Paraméter 1"="", "Paraméter 2"="", "Paraméter 3"="", "Paraméter 4"="", "Paraméter 5"="", "Eredmény"=""}, "Min"="", "Max"="", "Aktív?"=FALSE, "Log?"=FALSE, "Kiértékelés"=FALSE, "Etalon 1 exp"=FALSE, "Etalon 2 exp"=FALSE, "Etalon 3 exp"=FALSE, "Etalon 4 exp"=FALSE, "Etalon 5 exp"=FALSE}  # Teszt cluster
            n119 = Variant To Data(error in=w286, type=w292, Variant=w287) -> (data=w293:T9, error out=w290:errorcluster)
            n120 = Unbundle By Name(w293) -> ("Data"=w291:variant)
            n121 = Variant To Data(error in=w290, type=w289, Variant=w291) -> (data=w279:T7, error out=w276:errorcluster)
            n122 = call "AI data read single.vi"("error in (no error)"=w276, "Numeric"=Enum_AI."UISOL" ("Message"), "Message Queues in"=w266) -> ("error out"=w268:errorcluster, "Array"=w263:dbl[])  [unwired: 7 in]
            n123 = call-poly <vilib>:"Mean.vi"("X"=w263) -> ("mean"=w260:dbl)  [unwired: 1 out]
            n124 = call "AI data read single.vi"("error in (no error)"=w268, "Numeric"=Enum_AI."U48" ("Message"), "Message Queues in"=w266) -> ("error out"=w267:errorcluster, "Array"=w264:dbl[])  [unwired: 7 in]
            n125 = call-poly <vilib>:"Mean.vi"("X"=w264) -> ("mean"=w257:dbl)  [unwired: 1 out]
            n126 = Unbundle By Name(w279) -> ("Min"=w278:string)
            n127 = Fract/Exp String To Number(string=w278) -> (number=w261:dbl)  [unwired: 3 in, 1 out]
            n128 = Divide(x=w257, y=0.176 ("Im")) -> (x/y=w259:dbl)
            n129 = Less?(x=w260, y=w261) -> (x < y?=w277:bool)
            n130 = call "Rszig számítás.vi"("UIsol"=w261, "U48"=w259) -> ("Rszig"=w271:dbl)  [unwired: 9 in]
            n131 = call "Rszig számítás.vi"("UIsol"=w260, "U48"=w259) -> ("Rszig"=w262:dbl)  [unwired: 9 in]
            n132 = Divide(x=w262, y=1000000.0) -> (x/y=w274:dbl)
            n133 = Divide(x=w271, y=1000000.0) -> (x/y=w272:dbl)
            n134 = Unbundle By Name(w266) -> ("Engine"=w281:refnum<queue>)
            n135 = Number To Fractional String(number=w274) -> (F-format string=w280:string)  [unwired: 3 in]
            n136 = Number To Fractional String(number=w272) -> (F-format string=w275:string)  [unwired: 3 in]
            n137 = Bundle By Name(cluster=w279, "Command.Eredmény"=w280, "Kiértékelés"=w277, "Min"=w275) -> (w284:T7)
            n138 = Bundle By Name(cluster=w293, "Data"=w284) -> (w282:T9)
            n139 = Unbundle By Name(w282) -> ("Callback"=w283:string)
            n140 = call-poly "Enqueue Message.vi"("error in (no error)"=w267, "Message Data"=w282, "Message"=w283, "Message Queue"=w281) -> ("error out"=w288:errorcluster)  [unwired: 6 in, 1 out]
          }
          frame "DATAPROC Current Adj" {
            w322 = T9 {"Thread ID"=0, "Callback"="", "Data"=variant, "Error"={"status"=FALSE, "code"=0, "source"=""}}  # Message
            w319 = T7 {"Thread ID"=0.0, "Mérésszám"="", "Mérés/Utasítás"="", "Command"={"Parancs"="", "Paraméter 1"="", "Paraméter 2"="", "Paraméter 3"="", "Paraméter 4"="", "Paraméter 5"="", "Eredmény"=""}, "Min"="", "Max"="", "Aktív?"=FALSE, "Log?"=FALSE, "Kiértékelés"=FALSE, "Etalon 1 exp"=FALSE, "Etalon 2 exp"=FALSE, "Etalon 3 exp"=FALSE, "Etalon 4 exp"=FALSE, "Etalon 5 exp"=FALSE}  # Teszt cluster
            # "0 -> NTC\n1 -> R\n2 -> dU"
            n141 = Variant To Data(error in=w317, type=w322, Variant=w318) -> (data=w312:T9, error out=w320:errorcluster)
            n142 = Unbundle By Name(w312) -> ("Data"=w321:variant)
            n143 = Variant To Data(error in=w320, type=w319, Variant=w321) -> (data=w300:T7, error out=w315:errorcluster)
            n144 = Unbundle By Name(w300) -> ("Command.Paraméter 1"=w313:string)
            n145 = Unbundle By Name(w300) -> ("Command.Paraméter 2"=w301:string)
            n146 = Decimal String To Number(string=w313) -> (number=w307:i32)  [unwired: 2 in, 1 out]
            n147 = Decimal String To Number(string=w301) -> (number=w296:i32)  [unwired: 2 in, 1 out]
            n148 = case shown="0, Default" w307 {
              tunnel: w305 -> [w333 w346 w359]
              tunnel: w295 -> [w326 w339 w352]
              tunnel: [w325 w338 w351] -> w294
              frame 0, Default {
                n149 = Unbundle By Name(w333) -> ("DAQ"=w332:refnum<queue>)
                n150 = Bundle("Enum"=Enum_DO."NTC mérés relé", FALSE) -> (w336:cluster{"Enum":T6, bool})  [unwired: 1 in]
                n151 = Unbundle By Name(w326) -> ("UCTRL Cluster.UCTRL NTC"=w325:dbl)
                n152 = call-poly "Enqueue Message.vi"("Message Data"=w336, "Message"="Write DO Single", "Message Queue"=w332) -> ("dup Message Queue"=w327:refnum<queue>)  [unwired: 7 in, 1 out]
                n153 = Bundle("Enum"=Enum_DO."200mA relé", FALSE) -> (w329:cluster{"Enum":T6, bool})  [unwired: 1 in]
                n154 = call-poly "Enqueue Message.vi"("Message Data"=w329, "Message"="Write DO Single", "Message Queue"=w327) -> ()  [unwired: 7 in, 2 out]
              }
              frame 1 {
                n155 = Unbundle By Name(w346) -> ("DAQ"=w345:refnum<queue>)
                n156 = Bundle("Enum"=Enum_DO."R mérés relé", FALSE) -> (w349:cluster{"Enum":T6, bool})  [unwired: 1 in]
                n157 = call-poly "Enqueue Message.vi"("Message Data"=w349, "Message"="Write DO Single", "Message Queue"=w345) -> ("dup Message Queue"=w340:refnum<queue>)  [unwired: 7 in, 1 out]
                n158 = Unbundle By Name(w339) -> ("UCTRL Cluster.UCTRL R"=w338:dbl)
                n159 = Bundle("Enum"=Enum_DO."200mA relé", FALSE) -> (w342:cluster{"Enum":T6, bool})  [unwired: 1 in]
                n160 = call-poly "Enqueue Message.vi"("Message Data"=w342, "Message"="Write DO Single", "Message Queue"=w340) -> ()  [unwired: 7 in, 2 out]
              }
              frame 2 {
                n161 = Unbundle By Name(w359) -> ("DAQ"=w358:refnum<queue>)
                n162 = Bundle("Enum"=Enum_DO."R mérés relé", FALSE) -> (w362:cluster{"Enum":T6, bool})  [unwired: 1 in]
                n163 = call-poly "Enqueue Message.vi"("Message Data"=w362, "Message"="Write DO Single", "Message Queue"=w358) -> ("dup Message Queue"=w353:refnum<queue>)  [unwired: 7 in, 1 out]
                n164 = Unbundle By Name(w352) -> ("UCTRL Cluster.UCTRL dU"=w351:dbl)
                n165 = Bundle("Enum"=Enum_DO."200mA relé", TRUE) -> (w355:cluster{"Enum":T6, bool})  [unwired: 1 in]
                n166 = call-poly "Enqueue Message.vi"("Message Data"=w355, "Message"="Write DO Single", "Message Queue"=w353) -> ()  [unwired: 7 in, 2 out]
              }
            }
            n167 = Unbundle By Name(w305) -> ("NI Analog"=w306:refnum<queue>)
            n168 = case shown="0, Default" w296 {
              tunnel: [0.0 ("UCtrl") w324] -> w297
              tunnel: w294 -> [_ w324]
              frame 0, Default {
              }
              frame 1 {
              }
            }
            n169 = Bundle By Name(cluster=w295, "I Adj Parameters.I Adj step"=0, "I Adj Parameters.Output"=1.0) -> (w309:T2)
            n170 = Wait (ms)(milliseconds to wait=u32 100) -> ()  [unwired: 1 out]
            n171 = Bundle(cluster=cluster{i32, "UCtrl":dbl} {0, "UCtrl"=0.0}, Enum_AO."UCTRL" ("Enum"), "UCtrl"=w297) -> (w302:cluster{i32, "UCtrl":dbl})
            n172 = call-poly "Enqueue Message.vi"("Message Data"=w302, "Message"="OUTPUT Analog Write", "Message Queue"=w306) -> ()  [unwired: 7 in, 2 out]
            n173 = call-poly "Enqueue Message.vi"("error in (no error)"=w315, "Message Data"=w312, "Message"="DATAPROC Current Adj Read", "Message Queue"=w314) -> ("error out"=w316:errorcluster)  [unwired: 6 in, 1 out]
          }
          frame "DATAPROC Current Adj Read" {
            w399 = T9 {"Thread ID"=0, "Callback"="", "Data"=variant, "Error"={"status"=FALSE, "code"=0, "source"=""}}  # Message
            w396 = T7 {"Thread ID"=0.0, "Mérésszám"="", "Mérés/Utasítás"="", "Command"={"Parancs"="", "Paraméter 1"="", "Paraméter 2"="", "Paraméter 3"="", "Paraméter 4"="", "Paraméter 5"="", "Eredmény"=""}, "Min"="", "Max"="", "Aktív?"=FALSE, "Log?"=FALSE, "Kiértékelés"=FALSE, "Etalon 1 exp"=FALSE, "Etalon 2 exp"=FALSE, "Etalon 3 exp"=FALSE, "Etalon 4 exp"=FALSE, "Etalon 5 exp"=FALSE}  # Teszt cluster
            # "0 -> NTC\n1 -> R\n2 -> dU"
            n174 = Variant To Data(error in=w394, type=w399, Variant=w395) -> (data=w389:T9, error out=w397:errorcluster)
            n175 = Unbundle By Name(w389) -> ("Data"=w398:variant)
            n176 = Variant To Data(error in=w397, type=w396, Variant=w398) -> (data=w391:T7, error out=w371:errorcluster)
            n177 = Unbundle By Name(w391) -> ("Command.Paraméter 1"=w390:string)
            n178 = Decimal String To Number(string=w390) -> (number=w367:i32)  [unwired: 2 in, 1 out]
            n179 = case shown="0, 1, Default" w367 {
              tunnel: [Enum_AI."URref" ("Message") Enum_AI."dUref" ("Message")] -> w366
              frame 0, 1, Default {
              }
              frame 2 {
              }
            }
            n180 = case shown="0, Default" w367 {
              tunnel: w374 -> [w414 w417 w420]
              tunnel: [w413 w416 w419] -> w384
              tunnel: [1e-05 1e-05 0.0005] -> w377
              frame 0, Default {
                n181 = Unbundle By Name(w414) -> ("I Adj Parameters.Vr NTC"=w413:dbl)
              }
              frame 1 {
                n182 = Unbundle By Name(w417) -> ("I Adj Parameters.Vr R"=w416:dbl)
              }
              frame 2 {
                n183 = Unbundle By Name(w420) -> ("I Adj Parameters.Vr dU"=w419:dbl)
              }
            }
            n184 = call "AI data read single.vi"("error in (no error)"=w371, "Numeric"=w366, "Message Queues in"=w370) -> ("error out"=w369:errorcluster, "Array"=w368:dbl[])  [unwired: 7 in]
            n185 = call "dblvector_filtave.vi"("Eldobandó [%]"=40.0, "Mérési adatok"=w368) -> ("Szûrt átlag"=w365:dbl)  [unwired: 9 in]
            n186 = Unbundle By Name(w374) -> ("I Adj Parameters.I Adj step"=w388:i32, "I Adj Parameters.Output"=w381:dbl)
            n187 = Divide(x=w384, y=w365) -> (x/y=w383:dbl)
            n188 = Subtract(x=w384, y=w365) -> (x-y=w382:dbl)
            n189 = Absolute Value(x=w383) -> (abs(x)=w380:dbl)
            n190 = Absolute Value(x=w382) -> (abs(x)=w378:dbl)
            n191 = Less?(x=w378, y=w377) -> (x < y?=w372:bool)
            n192 = Increment(x=w388) -> (x+1=w386:i32)
            n193 = Multiply(x=w381, y=w380) -> (x*y=w376:dbl)
            n194 = Greater Or Equal?(x=w386, y=50) -> (x >= y?=w375:bool)
            n195 = Compound Arithmetic op=OR(w375, w372) -> (w379:bool)
            n196 = case shown="True" w379 {
              tunnel: [w406 w411] -> w393
              tunnel: w369 -> [w405 w410]
              tunnel: w392 -> [w404 w409]
              tunnel: w389 -> [w403 w408]
              frame False {
                n197 = call-poly "Enqueue Message.vi"("error in (no error)"=w405, "Message Data"=w403, "Message"="DATAPROC Current Adj Setup", "Message Queue"=w404) -> ("error out"=w406:errorcluster)  [unwired: 6 in, 1 out]
              }
              frame True {
                n198 = call-poly "Enqueue Message.vi"("error in (no error)"=w410, "Message Data"=w408, "Message"="DATAPROC Current Adj End", "Message Queue"=w409) -> ("error out"=w411:errorcluster)  [unwired: 6 in, 1 out]
              }
            }
            n199 = Bundle By Name(cluster=w374, "I Adj Parameters.I Adj step"=w386, "I Adj Parameters.Adj Failed"=w375, "I Adj Parameters.Output"=w376) -> (w373:T2)
            n200 = Wait (ms)(milliseconds to wait=u32 1 ("milliseconds to wait 2")) -> ()  [unwired: 1 out]
          }
          frame "DATAPROC Current Adj Setup" {
            w431 = 10.0 ("x")
            w432 = 0.001 ("y")
            w448 = T9 {"Thread ID"=0, "Callback"="", "Data"=variant, "Error"={"status"=FALSE, "code"=0, "source"=""}}  # Message
            w445 = T7 {"Thread ID"=0.0, "Mérésszám"="", "Mérés/Utasítás"="", "Command"={"Parancs"="", "Paraméter 1"="", "Paraméter 2"="", "Paraméter 3"="", "Paraméter 4"="", "Paraméter 5"="", "Eredmény"=""}, "Min"="", "Max"="", "Aktív?"=FALSE, "Log?"=FALSE, "Kiértékelés"=FALSE, "Etalon 1 exp"=FALSE, "Etalon 2 exp"=FALSE, "Etalon 3 exp"=FALSE, "Etalon 4 exp"=FALSE, "Etalon 5 exp"=FALSE}  # Teszt cluster
            n201 = Variant To Data(error in=w443, type=w448, Variant=w444) -> (data=w440:T9, error out=w446:errorcluster)
            n202 = Unbundle By Name(w440) -> ("Data"=w447:variant)
            n203 = Variant To Data(error in=w446, type=w445, Variant=w447) -> (error out=w427:errorcluster)  [unwired: 1 out]
            n204 = Unbundle By Name(w423) -> ("I Adj Parameters.Output"=w430:dbl)
            n205 = Greater?(x=w430, y=w432) -> (0:w433:bool)
            n206 = Select(t=w430, s=w433, f=w432) -> (s? t:f=w429:dbl)
            n207 = Unbundle By Name(w439) -> ("NI Analog"=w438:refnum<queue>)
            n208 = Less?(x=w431, y=w429) -> (x < y?=w434:bool)
            n209 = Select(t=w431, s=w434, f=w429) -> (s? t:f=w421:dbl)
            n210 = Bundle(cluster=cluster{i32, "UCtrl":dbl} {0, "UCtrl"=0.0}, Enum_AO."UCTRL" ("Enum"), "UCtrl"=w421) -> (w435:cluster{i32, "UCtrl":dbl})
            n211 = call-poly "Enqueue Message.vi"("error in (no error)"=w427, "Message Data"=w435, "Message"="OUTPUT Analog Write", "Message Queue"=w438) -> ("error out"=w426:errorcluster)  [unwired: 6 in, 1 out]
            n212 = Bundle By Name(cluster=w423, "I Adj Parameters.Output"=w421) -> (w422:T2)
            n213 = Wait (ms)(milliseconds to wait=u32 41) -> ()  [unwired: 1 out]
            n214 = call-poly "Enqueue Message.vi"("error in (no error)"=w426, "Message Data"=w440, "Message"="DATAPROC Current Adj Read", "Message Queue"=w441) -> ("error out"=w442:errorcluster)  [unwired: 6 in, 1 out]
          }
          frame "DATAPROC Current Adj End" {
            w477 = T9 {"Thread ID"=0, "Callback"="", "Data"=variant, "Error"={"status"=FALSE, "code"=0, "source"=""}}  # Message
            w474 = T7 {"Thread ID"=0.0, "Mérésszám"="", "Mérés/Utasítás"="", "Command"={"Parancs"="", "Paraméter 1"="", "Paraméter 2"="", "Paraméter 3"="", "Paraméter 4"="", "Paraméter 5"="", "Eredmény"=""}, "Min"="", "Max"="", "Aktív?"=FALSE, "Log?"=FALSE, "Kiértékelés"=FALSE, "Etalon 1 exp"=FALSE, "Etalon 2 exp"=FALSE, "Etalon 3 exp"=FALSE, "Etalon 4 exp"=FALSE, "Etalon 5 exp"=FALSE}  # Teszt cluster
            # "0 -> NTC\n1 -> R\n2 -> dU"
            n215 = Variant To Data(error in=w471, type=w477, Variant=w472) -> (data=w478:T9, error out=w475:errorcluster)
            n216 = Unbundle By Name(w478) -> ("Data"=w476:variant)
            n217 = Variant To Data(error in=w475, type=w474, Variant=w476) -> (data=w469:T7, error out=w457:errorcluster)
            n218 = Unbundle By Name(w456) -> ("I Adj Parameters.Output"=w462:dbl, "I Adj Parameters.Adj Failed"=w463:bool)
            n219 = Unbundle By Name(w469) -> ("Command.Paraméter 1"=w468:string)
            n220 = Decimal String To Number(string=w468, default (0L)=0 ("y")) -> (number=w466:i32)  [unwired: 1 in, 1 out]
            n221 = case shown="False" w463 {
              tunnel: w466 -> [w501 w515]
              tunnel: ["Adjust Success" ("Command.Eredmény") w511] -> w465
              tunnel: [TRUE FALSE] -> w464
              tunnel: w462 -> [w498 _]
              tunnel: w456 -> [w497 w516]
              tunnel: [w496 w516] -> w455
              frame False {
                n222 = case shown="0, Default" w501 {
                  tunnel: w498 -> [w504 w507 w510]
                  tunnel: w497 -> [w503 w506 w509]
                  tunnel: [w502 w505 w508] -> w496
                  frame 0, Default {
                    n223 = Bundle By Name(cluster=w503, "UCTRL Cluster.UCTRL NTC"=w504) -> (w502:T2)
                  }
                  frame 1 {
                    n224 = Bundle By Name(cluster=w506, "UCTRL Cluster.UCTRL R"=w507) -> (w505:T2)
                  }
                  frame 2 {
                    n225 = Bundle By Name(cluster=w509, "UCTRL Cluster.UCTRL dU"=w510) -> (w508:T2)
                  }
                }
              }
              frame True {
                n226 = Number To Decimal String(number=w515) -> (decimal integer string=w512:string)  [unwired: 1 in]
                n227 = call <vilib>:"Space Constant.vi"() -> ("String"=w513:string)
                n228 = Concatenate Strings("Adjust Failed" ("Command.Eredmény"), w513, w512) -> (w511:string)
              }
            }
            n229 = Unbundle By Name(w454) -> ("DAQ"=w453:refnum<queue>)
            n230 = disable-structure shown="Disabled" {
              disable-tunnel: w457 -> [w494 w495]
              disable-tunnel: w453 -> [w493 _]
              disable-tunnel: [w490 w495] -> w449
              frame Disabled {
                w481 = FALSE
                w480 = "Write DO Single" ("Message")
                n231 = Bundle("Enum"=Enum_AI."U48", w481) -> (w484:cluster{"Enum":T5, bool})  [unwired: 1 in]
                n232 = call-poly "Enqueue Message.vi"("error in (no error)"=w494, "Message Data"=w484, "Message"=w480, "Message Queue"=w493) -> ("error out"=w483:errorcluster, "dup Message Queue"=w485:refnum<queue>)  [unwired: 6 in]
                n233 = Bundle("Enum"=Enum_AI."URref", w481) -> (w488:cluster{"Enum":T5, bool})  [unwired: 1 in]
                n234 = call-poly "Enqueue Message.vi"("error in (no error)"=w483, "Message Data"=w488, "Message"=w480, "Message Queue"=w485) -> ("error out"=w486:errorcluster, "dup Message Queue"=w487:refnum<queue>)  [unwired: 6 in]
                n235 = Bundle("Enum"=Enum_AI."URref", w481) -> (w492:cluster{"Enum":T5, bool})  [unwired: 1 in]
                n236 = call-poly "Enqueue Message.vi"("error in (no error)"=w486, "Message Data"=w492, "Message"=w480, "Message Queue"=w487) -> ("error out"=w490:errorcluster)  [unwired: 6 in, 1 out]
              }
              frame Enabled {
              }
            }
            n237 = Bundle By Name(cluster=w469, "Command.Eredmény"=w465, "Kiértékelés"=w464) -> (w452:T7)
            n238 = Unbundle By Name(w454) -> ("Engine"=w470:refnum<queue>)
            n239 = Bundle By Name(cluster=w478, "Data"=w452) -> (w450:T9)
            n240 = Unbundle By Name(w450) -> ("Callback"=w451:string)
            n241 = Bundle By Name(cluster=w455, "I Adj Parameters.I Adj step"=0, "I Adj Parameters.Output"=1.0, "I Adj Parameters.Adj Failed"=FALSE) -> (w461:T2)
            n242 = disable-structure shown="Disabled" {
              frame Disabled {
                n243 = Wait (ms)(milliseconds to wait=u32 100) -> ()  [unwired: 1 out]
              }
              frame Enabled {
              }
            }
            n244 = call-poly "Enqueue Message.vi"("error in (no error)"=w449, "Message Data"=w450, "Message"=w451, "Message Queue"=w470) -> ("error out"=w473:errorcluster)  [unwired: 6 in, 1 out]
          }
          frame "Abort" {
            n245 = Flush Queue(queue=w520, error in (no error)=w521) -> (error out=w518:errorcluster)  [unwired: 2 out]
          }
          frame "Error" {
            n246 = Unbundle By Name(w525) -> ("UI"=w530:refnum<queue>)
            n247 = call-poly "Enqueue Message.vi"("error in (no error)"=w523, "Message Data"=w524, "Message"="Error", "Message Queue"=w530) -> ("error out"=w532:errorcluster)  [unwired: 6 in, 1 out]
            n248 = call-poly "Enqueue Message.vi"("Priority Message? (F)"=TRUE, "error in (no error)"=w523, "Message"="Initiate Stop", "Message Queue"=w526) -> ("error out"=w531:errorcluster)  [unwired: 6 in, 1 out]
            n249 = Merge Errors(w532, w531) -> (w527:errorcluster)
          }
          frame "Initiate Stop" {
            n250 = call-poly "Enqueue Message.vi"("Priority Message? (F)"=TRUE, "error in (no error)"=w537, "Message"="Program Stop", "Message Queue"=w536) -> ("error out"=w538:errorcluster)  [unwired: 6 in, 1 out]
          }
          frame "Program Stop" {
            n251 = Flush Queue(queue=w550, error in (no error)=w540) -> (error out=w542:errorcluster)  [unwired: 2 out]
            n252 = Unbundle By Name(w543) -> ("Data Processor data"=w544:refnum<queue>)
            n253 = Flush Queue(queue=w544, error in (no error)=w540) -> (queue out=w545:refnum<queue>, error out=w546:errorcluster)  [unwired: 1 out]
            n254 = Release Queue(queue=w545, error in (no error)=w546) -> (error out=w547:errorcluster)  [unwired: 1 in, 2 out]
            n255 = Merge Errors(w547, w542) -> (w541:errorcluster)
          }
          frame Default {
            n256 = xnode "Error Ring"("parameter 0"=w551) -> ("error out"=w552:errorcluster)
          }
        }
      }
      frame True {
        n257 = disable-structure shown="Disabled" {
          disable-tunnel: w566 -> [w586 _]
          disable-tunnel: w565 -> [w580 w596]
          disable-tunnel: [w579 w596] -> w564
          disable-tunnel: w563 -> [w578 w595]
          disable-tunnel: [w577 w595] -> w562
          frame Disabled {
            w585 = T10 {"DAQmx Tasks Started"=FALSE, "Csatorna jellemzõk"=[], "Delta U Puffer Enable"=FALSE, "Delta U Puffer"=refnum, "URref"="", "UR"="", "UNTC"="", "UISOL"="", "TEMP"="", "dUref"="", "dU_"="", "UCTRL"="", "U48"="", "NI analog"=""}  # Analog data
            w594 = T12 {"NI-6221 Continuous Sample"={"Sensor"=0.0, "Uref"=0.0, "Temperature"=0.0, "Uisol"=0.0, "NTC"=0.0, "U48"=0.0, "U15"=0.0}, "Analog Result"={"Szenzor ellenállás"=0.0, "NTC ellenállás"=0.0, "Szigetelési ellenállás"=0.0, "Hõmérséklet"=0.0, "48V"=0.0, "15V"=0.0, "Elvárt NTC ellenállás"=0.0, "Semmi 3"=0.0, "Semmi 4"=0.0, "Számolt NTC hõmérséklet"=0.0}, "NI-6221 N Sample"={"URref"=[], "UR"=[], "UNTC"=[], "UISOL"=[], "TEMP"=[], "dUref"=[], "dU"=[], "U48"=[]}}  # NI Analog Input
            n258 = Unbundle By Name(w586) -> ("AI data"=w582:refnum<queue>)
            n259 = call "Preview Message.vi"("error in (no error)"=w580, "Message Queue"=w582) -> ("error out"=w583:errorcluster, "Message Data"=w584:variant)  [unwired: 5 in, 3 out]
            n260 = Variant To Data(error in=w583, type=w585, Variant=w584) -> (data=w569:T10, error out=w581:errorcluster)
            n261 = call "FIFO last element.vi"("error in (no error)"=w581, "Analog data"=w569) -> ("error out"=w587:errorcluster, "Last elements"=w588:dbl[])  [unwired: 6 in, 2 out]
            n262 = call <vilib>:"Clear Errors.vi"("error in (no error)"=w587) -> ("error out"=w579:errorcluster)  [unwired: 5 in, 1 out]
            n263 = Split 1D Array(array=w588, index=7) -> (first subarray=w592:dbl[], second subarray=w590:dbl[])
            n264 = Array To Cluster(array=w592) -> (cluster=w591:T14)
            n265 = Array To Cluster(array=w590) -> (cluster=w589:T15)
            n266 = Bundle By Name(cluster=w594, "NI-6221 Continuous Sample"=w591, "Analog Result"=w589) -> (w576:T12)
            n267 = Unbundle By Name(w576) -> ("Analog Result.Szenzor ellenállás"=w575:dbl, "Analog Result.NTC ellenállás"=w574:dbl, "Analog Result.Szigetelési ellenállás"=w573:dbl, "Analog Result.Hõmérséklet"=w572:dbl, "Analog Result.Elvárt NTC ellenállás"=w571:dbl, "Analog Result.Számolt NTC hõmérséklet"=w570:dbl)
            n268 = Unbundle By Name(w569) -> ("Delta U Puffer"=w568:refnum<queue>)
            n269 = Bundle By Name(cluster=w578, "R Res"=w575, "NTC Res"=w574, "Insulation Res"=w573, "Temperature"=w572, "NTC Exp Res"=w571, "NTC Calc Temp"=w570, "Delta U Puffer"=w568) -> (w577:T2)
          }
          frame Enabled {
          }
        }
      }
    }
    n270 = call "Error Handler - Message Handling Loop.vi"("error in (no error)"=w11, "Message Queue"=w7) -> ("dup error in"=w12:errorcluster, "dup Message Queue"=w9:refnum<queue>)  [unwired: 8 in]
  }
  "error out" <- w6
  "Message Queue" <- w2
